vi "arraymenuring.vi"(1 "Array In":u16[](array[ring]) items=["A", "B", "C"]) -> (0 "Array Out":u16[](array[ring]) items=["A", "B", "C"])   [LabVIEW 2010]
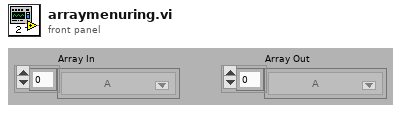
[diagram p1: front panel]
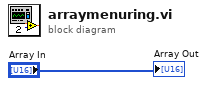
[diagram p0: block diagram]
diagram:
  "Array Out" <- "Array In"
